vi "UDCPauseNetworkActivity.vi"(8 "Error In":errorcluster, 11 "Pause Network Activity":bool) -> (0 "Error Out":errorcluster)   [LabVIEW 2020, in "niceiplib.lvlib"]
doc: "This API puases the network activity until it is unpaused."
uses:
  <vilib>/UDC/niceiplib.lvlib
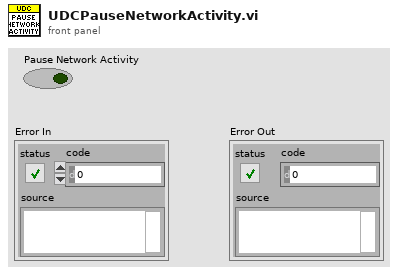
[diagram p1: front panel]
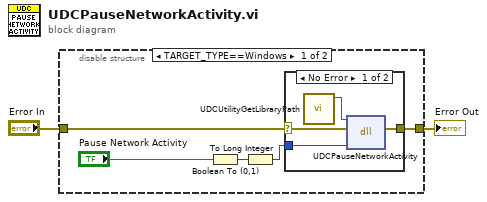
[diagram p0: block diagram]
diagram:
  n1 = disable-structure shown="TARGET_TYPE==Windows" {
    disable-tunnel: [w4 w13] -> w2
    disable-tunnel: "Error In" -> [w3 w13]
    frame condition #0 (active) {
      n2 = Boolean To (0,1)(Boolean="Pause Network Activity") -> (0, 1=w7:i16)
      n3 = To Long Integer(number=w7) -> (32bit integer=w6:i32)
      n4 = case shown="No Error" w3 {
        selector: w3 -> [w9 w12]
        tunnel: w6 -> [w11 _]
        tunnel: [w10 w12] -> w4
        frame No Error {
          n5 = call <vilib>:"UDCUtilityGetLibraryPath.vi"() -> ("Library Path"=w8:path)  [unwired: 11 in]
          n6 = dll-call lib="C:/2013LabVIEWCode/dist/vi.lib/UDC/niceiplib.*" fn="UDCPauseNetworkActivity"(path in=w8, error in=w9, "pause"=w11) -> (error out=w10:errorcluster)  [unwired: 3 in, 1 out]
        }
        frame Error {
        }
      }
    }
    frame condition #1 {
    }
  }
  "Error Out" <- w2
